vi "PCI1220U位置模式.vi"(10 "Distance":dbl=10000.0, 11 "AxisHandle IN":u32) -> (2 "AbsSuccess":bool, 3 "AxisHandle OUT":u32)   [LabVIEW 2013]
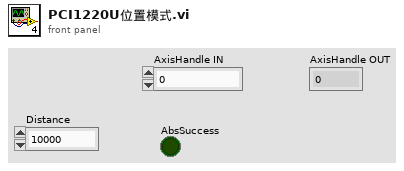
[diagram p1: front panel]
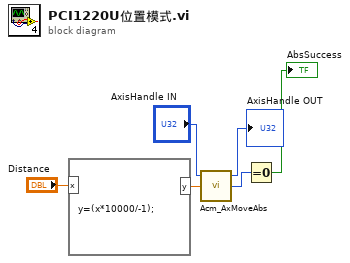
[diagram p0: block diagram]
diagram:
  n1 = formula code="y=(x*10000/-1);"("x"="Distance") -> ("y"=w3:dbl)
  n2 = call <userlib>:"Acm_AxMoveAbs.vi"("Position"=w3, "AxisHandle"="AxisHandle IN") -> ("ReturnValue"=w1:u32, "AxisHandle"=→"AxisHandle OUT":u32)  [unwired: 1 in, 1 out]
  n3 = Equal To 0?(x=w1) -> (x = 0?=→"AbsSuccess":bool)
